vi "CANdle_open.vi"(8 "error in":errorcluster, 10 "CANbus Name":string="rio", 11 "Device ID":u8) -> (0 "error out":errorcluster, 3 "DeviceReference 2":T1)   [LabVIEW 2025]
uses:
  <vilib>/Rock Robotics/WPI/ThirdParty/Phoenix6/DeviceReference.ctl
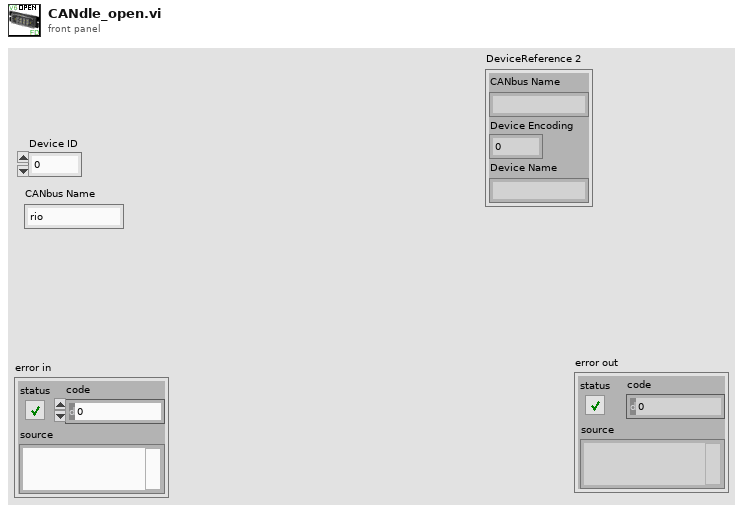
[diagram p1: front panel]
types:
  T1 = typedef "DeviceReference.ctl" = cluster{"CANbus Name":string, "Device Encoding":u32, "Device Name":string}
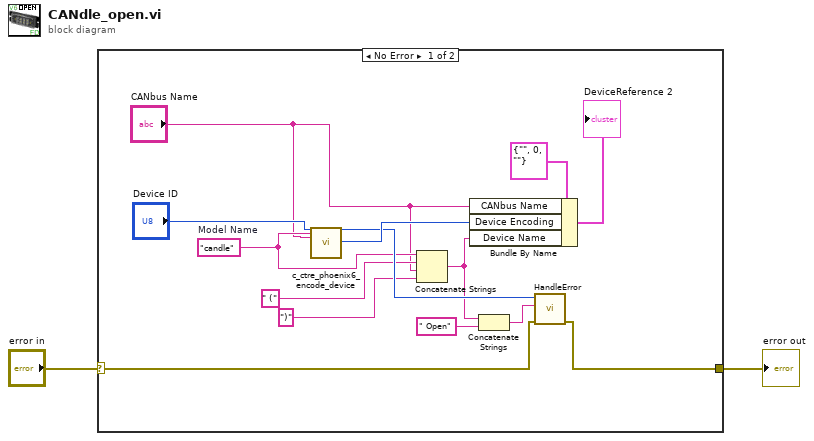
[diagram p0: block diagram]
diagram:
  n1 = case shown="No Error" "error in" {
    selector: "error in" -> [w11 w17]
    tunnel: [w10 w17] -> w1
    frame No Error {
      w7 = "candle"  # Model Name
      n2 = call <vilib>:"c_ctre_phoenix6_encode_device.vi"("Numeric 2"="Device ID", "String 2"=w7, "String 4"="CANbus Name") -> ("Numeric"=w12:i32, "Numeric 3"=w13:u32)  [unwired: 21 in, 2 out]
      n3 = Concatenate Strings(w7, " (" ("string"), "CANbus Name", ")" ("string")) -> (w3:string)
      n4 = Bundle By Name(cluster=T1 {"CANbus Name"="", "Device Encoding"=0, "Device Name"=""} ("DeviceReference"), "CANbus Name"="CANbus Name", "Device Encoding"=w13, "Device Name"=w3) -> (→"DeviceReference 2":T1)
      n5 = Concatenate Strings(w3, " Open" ("string")) -> (w8:string)
      n6 = call <vilib>:"HandleError.vi"("error in"=w11, "origin"=w8, "Status"=w12) -> ("error out"=w10:errorcluster)  [unwired: 8 in]
    }
    frame Error {
    }
  }
  "error out" <- w1
